vi "NQ Computer Metadata.vi"(8 "error in (no error)":errorcluster) -> (0 "error out":errorcluster)   [LabVIEW 2020]
uses:
  Type Definitions/Enum - Metadata.ctl
  Type Definitions/Payload Class.ctl
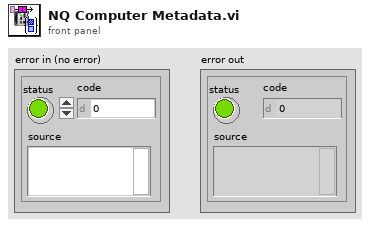
[diagram p1: front panel]
types:
  T1 = typedef "Payload Class.ctl" = enum16{"System State", "Parameters", "Metadata", "Software Monitor", "Data", "Commands"}
  T2 = typedef "Enum - Metadata.ctl" = enum16{"Computer Metadata", "Computer Resources", "RT Image Metadata", "Startup Settings", "Telemetry Recorder Status"}
  T3 = typedef "Computer Metadata.ctl" = cluster{"Kernel Name":string, "Node Name":string, "Kernel Release":string, "Kernel Version":string, "Machine":string, "Operating System":string}
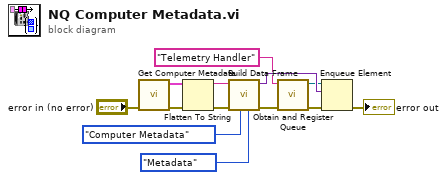
[diagram p0: block diagram]
diagram:
  n1 = call "Get Computer Metadata.vi"("error in (no error)"="error in (no error)") -> ("error out"=w5:errorcluster, "Computer Metadata"=w1:T3)  [unwired: 9 in]
  n2 = Flatten To String(anything=w1, error in (no error)=w5) -> (data string=w2:string, error out=w6:errorcluster)  [unwired: 2 in, 1 out]
  n3 = call "Build Data Frame.vi"("Payload Class (Data)"=Payload_Class."Metadata", "Payload ID (0)"=Enum_-_Metadata."Computer Metadata", "error in (no error)"=w6, "Payload (Empty String)"=w2) -> ("error out"=w11:errorcluster, "Frame"=w9:variant)  [unwired: 6 in]
  n4 = call "Obtain and Register Queue.vi"("error in (no error)"=w11, "name (unnamed)"="Telemetry Handler") -> ("error out"=w12:errorcluster, "Queue Out"=w8:refnum<queue>)  [unwired: 6 in, 2 out]
  n5 = Enqueue Element(queue=w8, element=w9, error in (no error)=w12) -> (error out=→"error out":errorcluster)  [unwired: 1 in, 2 out]
